vi "CalcDivSubVi.vi"(9 "Focus, mm":dbl, 10 "Pixel size, um":dbl, 11 "Width, px":i32) -> (2 "Divergence, mrad":dbl, 3 "Width, um":dbl)   [LabVIEW 2017]
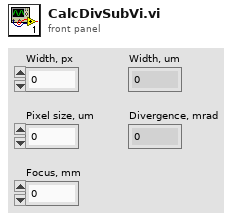
[diagram p1: front panel]
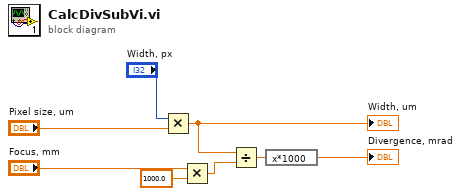
[diagram p0: block diagram]
diagram:
  n1 = Multiply(x="Width, px", y="Pixel size, um") -> (x*y=w6:dbl)
  "Width, um" <- w6
  n2 = Multiply(x="Focus, mm", y=1000.0) -> (x*y=w3:dbl)
  n3 = Divide(x=w6, y=w3) -> (x/y=w2:dbl)
  n4 = expression code="x*1000"(w2) -> (→"Divergence, mrad":dbl)
